vi "BNC555.evt call Run or Stop.vi"(0 "i ref in":refnum<vi>, 2 "Generator Instance":string="N/A", 3 "Start\\Stop":bool, 5 "error in (no error)":errorcluster) -> (14 "i ref out":refnum<vi>, 19 "error out":errorcluster)   [LabVIEW 2014, in "BNC555.lvlib"]
doc: "This VI sends a simple event call to the wired BNC555."
uses:
  BNC555.lvlib
  CS_Core/CSSystem/CoreLib/CoreLib.short 2 byte array.vi
  CS_Core/CSSystem/CoreLib/CoreLib.lvlib
  CS_Core/BaseProcess/BaseProcess.lvlib
panel:
  # "Run\nStop"
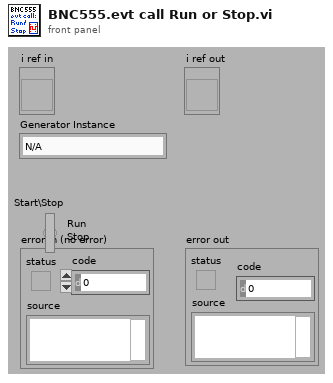
[diagram p1: front panel]
types:
  T1 = typedef "CoreDefs.rawDataType.ctl" = i8[]
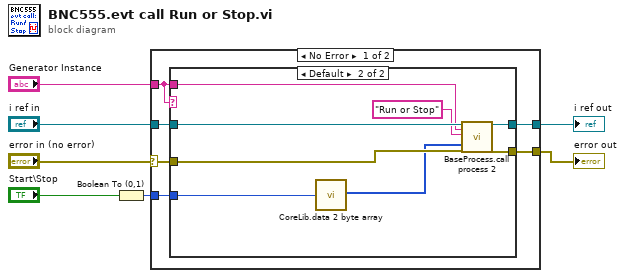
[diagram p0: block diagram]
diagram:
  n1 = Boolean To (0,1)(Boolean="Start\\Stop") -> (0, 1=w2:i16)
  n2 = case shown="No Error" "error in (no error)" {
    selector: "error in (no error)" -> [w10 w24]
    tunnel: [w13 w25] -> w6
    tunnel: [w12 w24] -> w5
    tunnel: "i ref in" -> [w11 w25]
    tunnel: "Generator Instance" -> [w9 _]
    tunnel: w2 -> [w8 _]
    frame No Error {
      n3 = case shown="Default" w9 {
        tunnel: [w15 w23] -> w13
        tunnel: [w14 w22] -> w12
        tunnel: w11 -> [w15 w21]
        tunnel: w9 -> [_ w20]
        tunnel: w10 -> [w14 w18]
        tunnel: w8 -> [_ w17]
        frame "N/A" {
        }
        frame Default {
          n4 = call-poly "CoreLib.data 2 byte array.vi"("i16"=w17) -> ("byteArray out"=w16:T1)  [unwired: 18 in]
          n5 = call "BaseProcess.call process 2.vi"("i ref in"=w21, "Object"=w20, "Selector"="Run or Stop", "Data"=w16, "error in (no error)"=w18) -> ("i ref out"=w23:refnum<vi>, "error out"=w22:errorcluster)  [unwired: 13 in]
        }
      }
    }
    frame Error {
    }
  }
  "error out" <- w5
  "i ref out" <- w6
